vi "Key Strokes Simulation_LV2012_NI Verified.vi"() -> ()   [LabVIEW 2020, in "MacroAssert.lvlib"]
doc: "This VI is an example that uses simulated Key Presses to type into a String control programmatically."
uses:
  MacroAssert.lvlib
panel:
  in  "Key Array":T1(array[cluster])=[{" Key"=16, "Action"=enum."Down", "Delay (ms)"=10}, {" Key"=72, "Action"=enum."Press", "Delay (ms)"=100}, {" Key"=16, "Action"=enum."Up", "Delay (ms)"=10}, {" Key"=69, "Action"=enum."Press", "Delay (ms)"=100}, {" Key"=76, "Action"=enum."Press", "Delay (ms)"=100}, {" Key"=76, "Action"=enum."Press", "Delay (ms)"=100}, {" Key"=79, "Action"=enum."Press", "Delay (ms)"=100}]
  in  "Output":string
  # "Overview: This VI is an example that uses simulated Key Presses to type into a String control programmatically.  \nRequirements: LabVIEW 2012 (or compatible)\nInstructions:\n1. Enter the keys in the Key Array control. It is what defines which keys are pressed and for how long.  Note that the shift key is pushed down and up in separate steps and that the alphabetical keys are pressed. This is equivalent to holding the shift key down while pressing\n'H', the result being an uppercase 'H'.\n2. Run this VI and 'Hello' will be programmatically typed in the Output box."
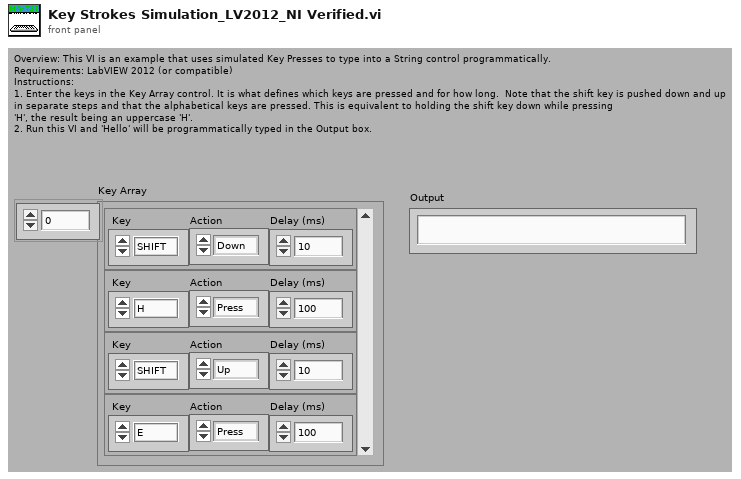
[diagram p1: front panel]
types:
  T1 = cluster{" Key":u8, "Action":enum16{"Press", "Up", "Down"}, "Delay (ms)":u32}[]
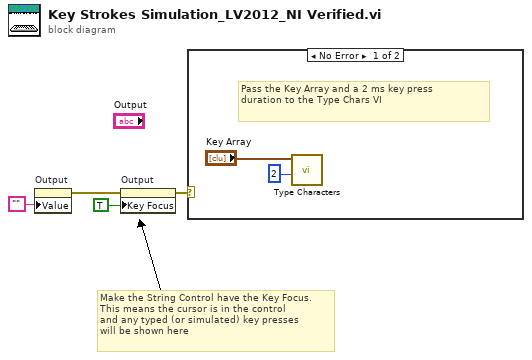
[diagram p0: block diagram]
diagram:
  # "Make the String Control have the Key Focus.\nThis means the cursor is in the control\nand any typed (or simulated) key presses\nwill be shown here"
  n1 = property on="Output" class="Str"("Value"="") -> (error out=w1:errorcluster)  [unwired: 2 in, 1 out]
  n2 = property on="Output" class="Str"(error in=w1, "Key Focus"=TRUE) -> (error out=w3:errorcluster)  [unwired: 1 in, 1 out]
  n3 = case shown="No Error" w3 {
    frame No Error {
      # "Pass the Key Array and a 2 ms key press\nduration to the Type Chars VI"
      n4 = call "Type Characters.vi"("Length of Key Press (ms)"=u32 2, "Key Array"="Key Array") -> ()  [unwired: 10 in]
    }
    frame Error {
    }
  }
